vi "AddHeader.vi"(8 "error in (no error)":errorcluster, 11 "LoggerPath":path) -> (0 "error out":errorcluster)   [LabVIEW 2021, in "Event Logger.lvlib"]
uses:
  Event Logger.lvlib
  <vilib>/Utility/file.llb/Write Delimited Spreadsheet (string).vi
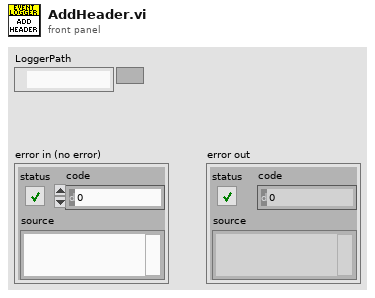
[diagram p1: front panel]
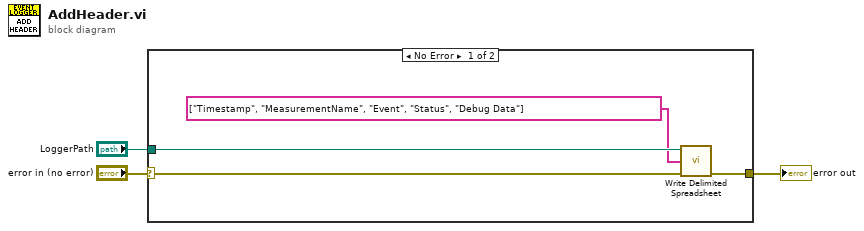
[diagram p0: block diagram]
diagram:
  n1 = case shown="No Error" "error in (no error)" {
    selector: "error in (no error)" -> [w4 w8]
    tunnel: "LoggerPath" -> [w7 _]
    tunnel: [w5 w8] -> w2
    frame No Error {
      n2 = call-poly <vilib>:"Write Delimited Spreadsheet.vi"("file path (dialog if empty)"=w7, "1D data"=string[] ["Timestamp", "MeasurementName", "Event", "Status", "Debug Data"] ("string"), "error in (no error)"=w4) -> ("error out"=w5:errorcluster)  [unwired: 11 in, 1 out]
    }
    frame Error {
    }
  }
  "error out" <- w2
